vi "READ CAN DATA.vi"(7 "Enum":T2=enum."GET", 8 "error in (no error)":errorcluster, 11 "CAN DATA":T1[](array[typedef])) -> (0 "error out":errorcluster, 3 "READ DATA OUT":T1[](array[typedef]))   [LabVIEW 2018]
uses:
  Controls/READ CAN DATA.ctl
  Controls/READ CAN CLUSTER.ctl
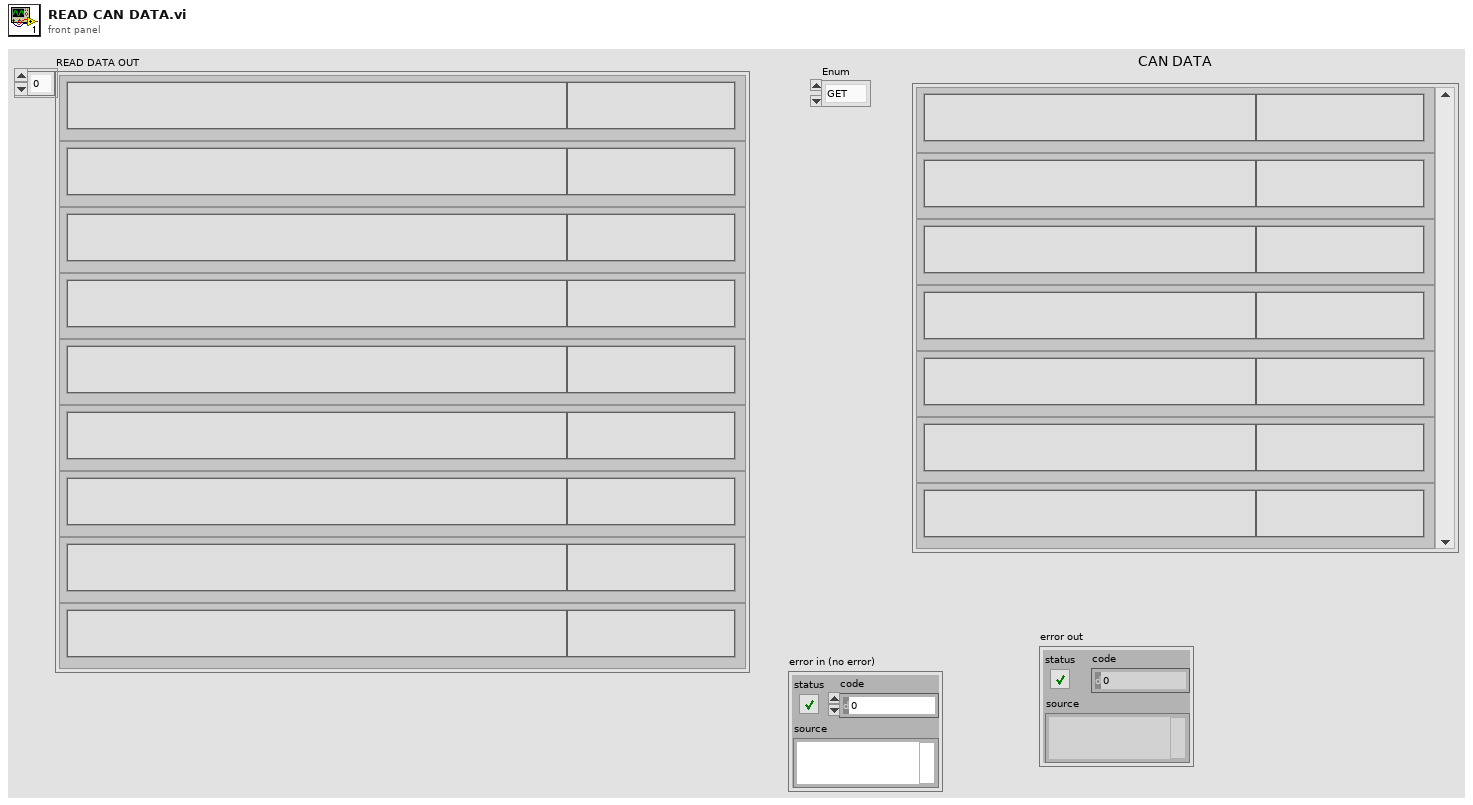
[diagram p1: front panel]
types:
  T1 = typedef "READ CAN CLUSTER.ctl" = cluster{"FUNCTION":string, "DATA":string}
  T2 = typedef "READ CAN DATA.ctl" = enum16{"SET", "GET"}
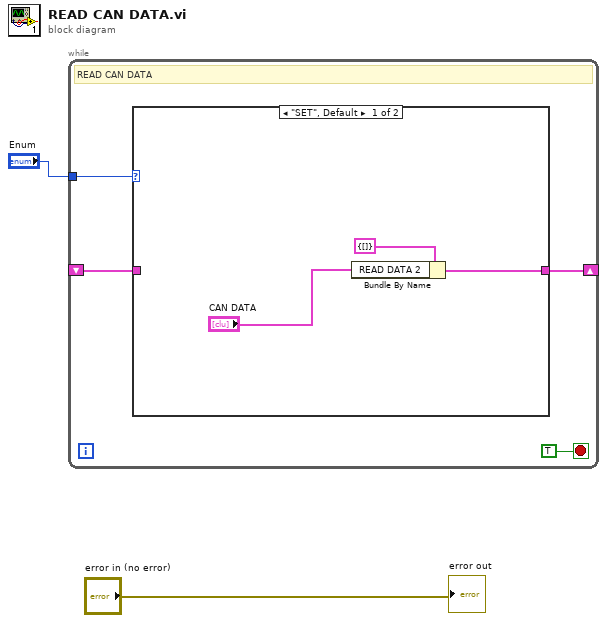
[diagram p0: block diagram]
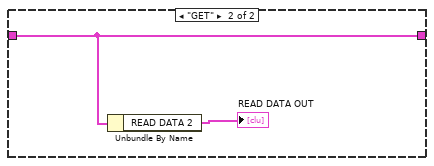
[diagram p2: hidden frame]
diagram:
  n1 = while {
    tunnel: "Enum" -> [w5]
    shift-right: [w4] -> _
    shift-left: _ -> [w3]
    stop <- TRUE stop-if-true
    # "READ CAN DATA"
    n2 = case shown="\"SET\", Default" w5 {
      tunnel: [w7 w11] -> w4
      tunnel: w3 -> [_ w11]
      frame "SET", Default {
        n3 = Bundle By Name(cluster=cluster{"READ DATA 2":T1[]} {"READ DATA 2"=[]}, "READ DATA 2"="CAN DATA") -> (w7:cluster{"READ DATA 2":T1[]})
      }
      frame "GET" {
        n4 = Unbundle By Name(w11) -> ("READ DATA 2"=→"READ DATA OUT":T1[])
      }
    }
  }
  "error out" <- "error in (no error)"
